vi "Set Packed Library Name.vi"(8 "error in (no error)":errorcluster, 10 "Packed library name":string, 11 "PPL in":refnum<class "NI_AB_API_PPL.lvclass">) -> (0 "error out":errorcluster, 3 "PPL out":refnum<class "NI_AB_API_PPL.lvclass">)   [LabVIEW 2020, in "NI_AB_API_PPL.lvclass"]
uses:
  <vilib>/AppBuilder/AB_API/PPL/NI_AB_API_PPL.lvclass
  e:/builds/penguin/labview/branches/2020/dev/dist/vi.lib/AppBuilder/AB_API/Build/NI_AB_API_Build.lvclass
  <vilib>/AppBuilder/AB_Classes/PackedLib/AB_PackedLibrary.lvclass
  e:/builds/penguin/labview/branches/2020/dev/dist/vi.lib/AppBuilder/AB_Classes/TargetFile/AB_Targetfile.lvclass
  e:/builds/penguin/labview/branches/2020/dev/dist/vi.lib/AppBuilder/AB_Classes/Build/AB_Build.lvclass
  <resource>/Framework/Providers/Common/provcom_StringGlobals.vi
  <vilib>/AppBuilder/AB_API/Build/NI_AB_API_Build.lvclass
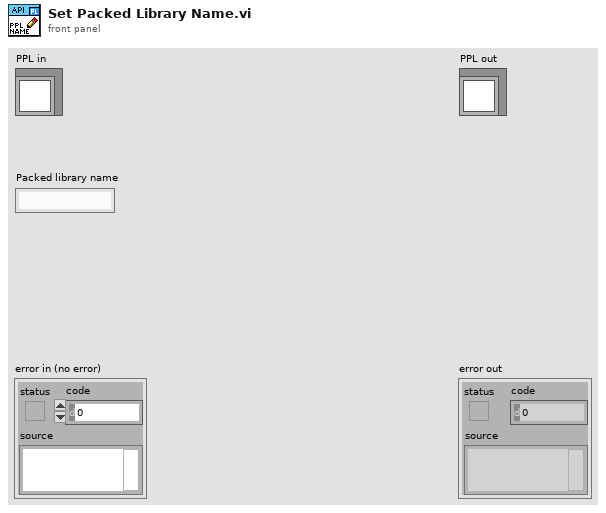
[diagram p1: front panel]
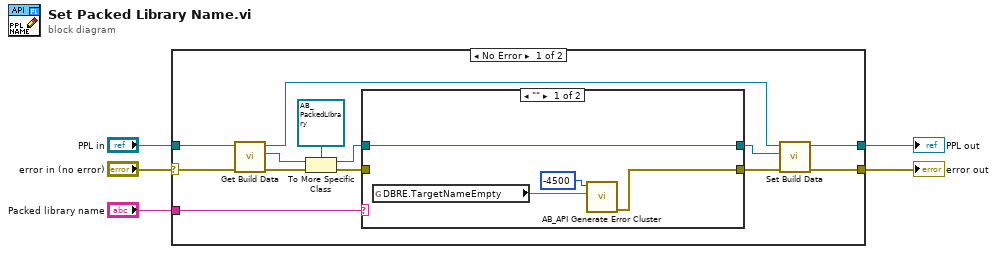
[diagram p0: block diagram]
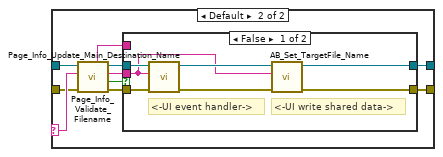
[diagram p2: hidden frame]
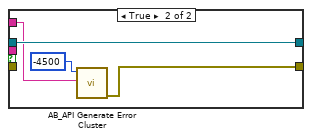
[diagram p3: hidden frame]
diagram:
  n1 = case shown="No Error" "error in (no error)" {
    selector: "error in (no error)" -> [w6 w45]
    tunnel: [w18 w45] -> w5
    tunnel: "PPL in" -> [w17 w44]
    tunnel: [w16 w44] -> w3
    tunnel: "Packed library name" -> [w15 _]
    frame No Error {
      n2 = call <vilib>:"Get Build Data.vi"("error in (no error)"=w6, "NI_AB_API_Build in"=w17) -> ("error out"=w14:errorcluster, "AB_Build.lvclass"=w8:refnum<class "AB_Build.lvclass">, "NI_AB_API_Build out"=w12:refnum<class "NI_AB_API_PPL.lvclass">)  [unwired: 7 in]
      n3 = To More Specific Class(target class=refnum<class "AB_PackedLibrary.lvclass"> refnum ("AB_PackedLibrary in"), reference=w8, error in=w14) -> (specific class reference=w7:refnum<class "AB_PackedLibrary.lvclass">, error out=w13:errorcluster)
      n4 = case shown="\"\"" w15 {
        selector: w15 -> [_ w28]
        tunnel: [w20 w32] -> w11
        tunnel: w13 -> [_ w25]
        tunnel: w7 -> [w19 w30]
        tunnel: [w19 w31] -> w10
        frame "" {
          n5 = global read "provcom_StringGlobals.vi" "DBRE.TargetNameEmpty"() -> (w21:string)
          n6 = call <vilib>:"AB_API Generate Error Cluster.vi"("Additional Message"=w21, "Code"=-4500) -> ("error out"=w20:errorcluster)  [unwired: 9 in]
        }
        frame Default {
          n7 = call-dynamic "Page_Info_Validate_Filename.vi"("error in (no error)"=w25, "Filename in"=w28, "AB_PackedLibrary in"=w30) -> ("error out"=w24:errorcluster, "hasInvalidCharacters"=w26:bool, "Filename out"=w27:string, "AB_PackedLibrary out"=w29:refnum<class "AB_PackedLibrary.lvclass">, "message"=w23:string)  [unwired: 4 in]
          n8 = case shown="False" w26 {
            tunnel: [w38 w42] -> w32
            tunnel: w24 -> [w36 _]
            tunnel: w29 -> [w35 w41]
            tunnel: [w39 w41] -> w31
            tunnel: w27 -> [w33 _]
            tunnel: w23 -> [_ w40]
            frame False {
              # "<-UI write shared data->"
              # "<-UI event handler->"
              n9 = call-dynamic "Page_Info_Update_Main_Destination_Name.vi"("error in (no error)"=w36, "destination name"=w33, "AB_Build in"=w35) -> ("error out"=w37:errorcluster, "AB_Build out"=w34:refnum<class "AB_PackedLibrary.lvclass">)  [unwired: 7 in]
              n10 = call <vilib>:"AB_Set_TargetFile_Name.vi"("error in (no error)"=w37, "Target filename"=w33, "TargetFile in"=w34) -> ("error out"=w38:errorcluster, "TargetFile out"=w39:refnum<class "AB_PackedLibrary.lvclass">)  [unwired: 7 in]
            }
            frame True {
              n11 = call <vilib>:"AB_API Generate Error Cluster.vi"("Additional Message"=w40, "Code"=-4500) -> ("error out"=w42:errorcluster)  [unwired: 9 in]
            }
          }
        }
      }
      n12 = call <vilib>:"Set Build Data.vi"("error in (no error)"=w11, "AB_Build.lvclass"=w10, "NI_AB_API_Build in"=w12) -> ("error out"=w18:errorcluster, "NI_AB_API_Build out"=w16:refnum<class "NI_AB_API_PPL.lvclass">)  [unwired: 7 in]
    }
    frame Error {
    }
  }
  "error out" <- w5
  "PPL out" <- w3
